vi "InitiateEventDisplay.vi"(6 "error in":errorcluster, 7 "colors":T1={"Frame color"=0, "Connectors color"=0, "Supports color"=0, "Bolts color"=0, "Scintillators color"=0, "Scintillator alpha"=0.5}, 8 "Scale":sgl, 9 "Path to detector WRL file":path) -> (0 "error out":errorcluster, 3 "Event Display Scene":refnum<vi>)   [LabVIEW 2016]
uses:
  <vilib>/picture/3D Picture Control/Object/Create Object (name).vi
  <vilib>/picture/3D Picture Control/NI_3D Picture Control.lvlib
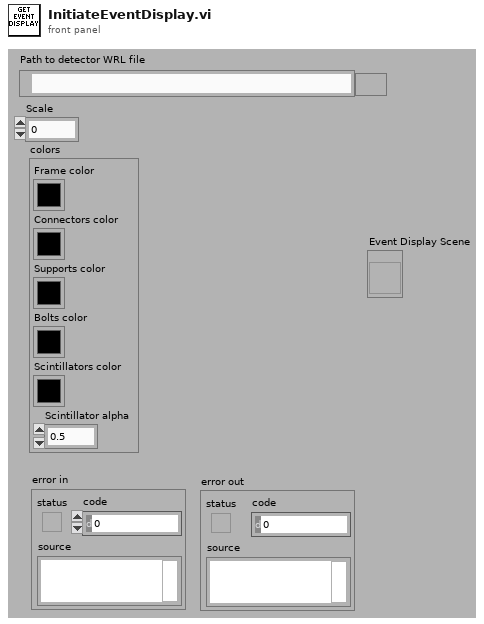
[diagram p1: front panel]
types:
  T1 = cluster{"Frame color":u32, "Connectors color":u32, "Supports color":u32, "Bolts color":u32, "Scintillators color":u32, "Scintillator alpha":sgl}
  T2 = enum16{"Normal Bin", "Opaque Bin", "Transparent Bin"}
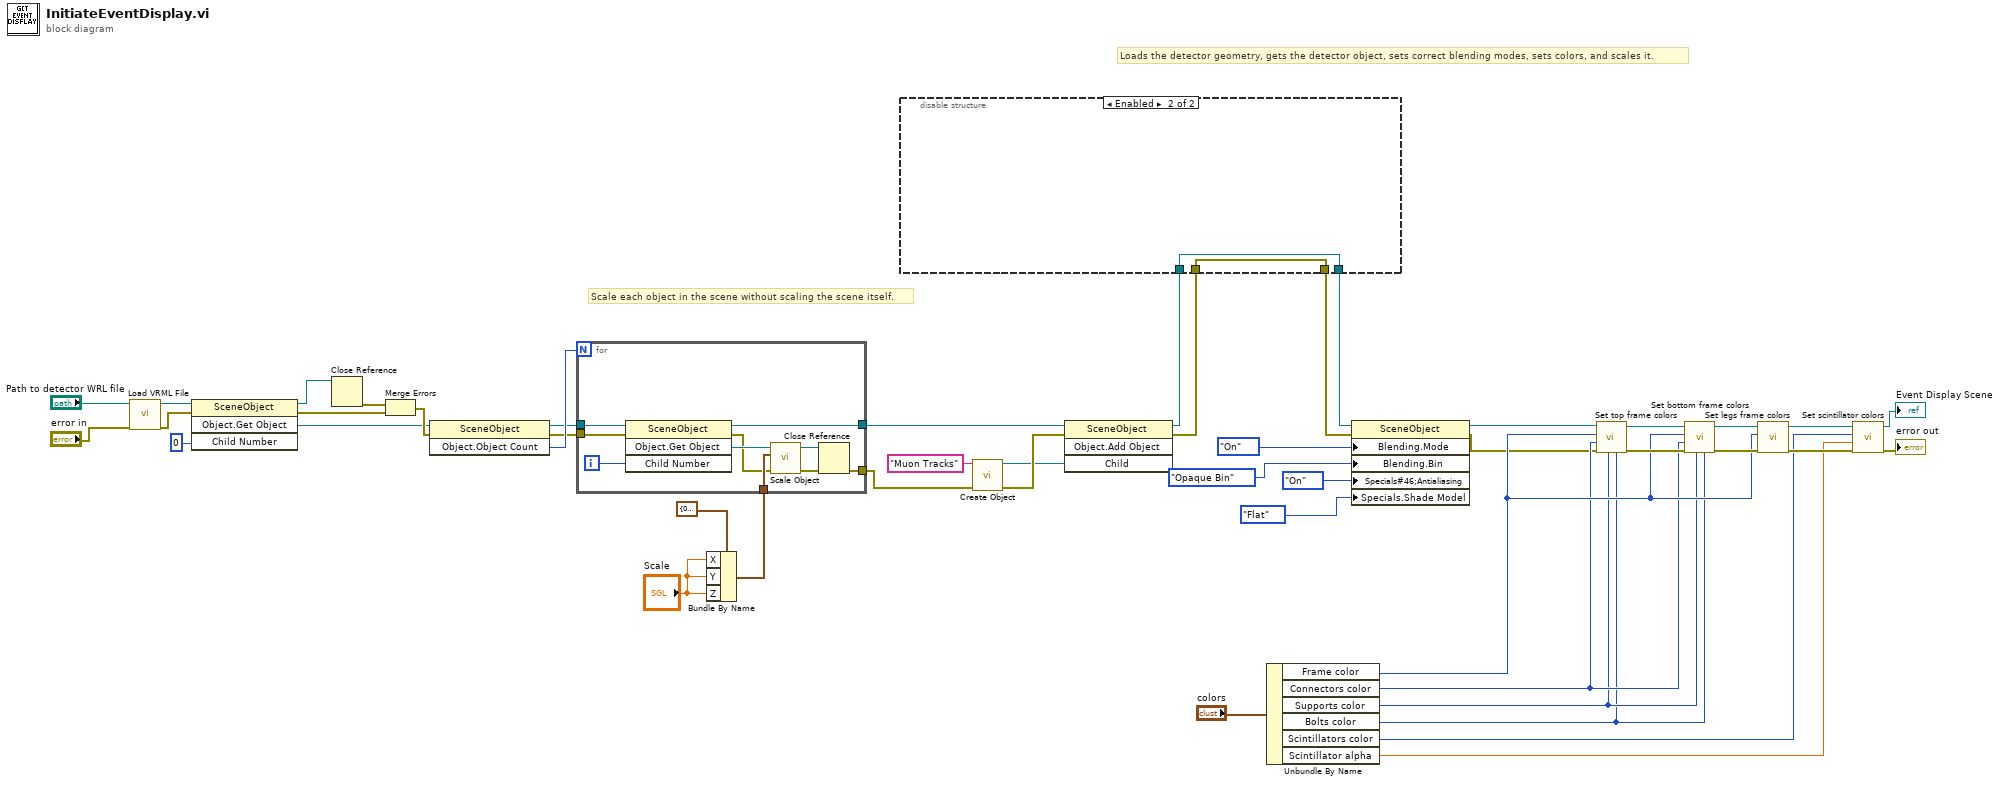
[diagram p0: block diagram]
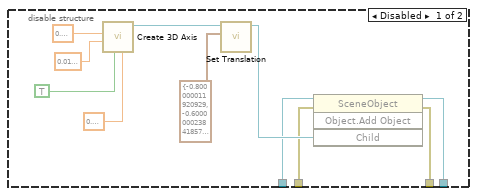
[diagram p2: hidden frame]
diagram:
  # "Scale each object in the scene without scaling the scene itself."
  # "Loads the detector geometry, gets the detector object, sets correct blending modes, sets colors, and scales it."
  n1 = call <vilib>:"Load VRML File.vi"("error in"="error in", "Path"="Path to detector WRL file") -> ("error out"=w26:errorcluster, "Scene:Read Scene File"=w45:refnum<vi>)  [unwired: 8 in]
  n2 = invoke class="SceneObject" method="Object.Get Object"(reference=w45, error in=w26, "Child Number"=0 ("index")) -> (reference out=w24:refnum<vi>, error out=w22:errorcluster, "Get Child"=w14:refnum<vi>)  [unwired: 1 in, 1 out]
  n3 = Close Reference(reference=w24) -> (error out=w23:errorcluster)  [unwired: 1 in]
  n4 = Merge Errors(w23, w22) -> (w15:errorcluster)
  n5 = invoke class="SceneObject" method="Object.Object Count"(reference=w14, error in=w15) -> (reference out=w12:refnum<vi>, error out=w11:errorcluster, "Child Count"=w13:i32)  [unwired: 1 in]
  n6 = Bundle By Name(cluster=cluster{"X":sgl, "Y":sgl, "Z":sgl} {"X"=0.0, "Y"=0.0, "Z"=0.0} ("Scale"), "X"="Scale", "Y"="Scale", "Z"="Scale") -> (w10:cluster{"X":sgl, "Y":sgl, "Z":sgl})
  n7 = for {
    N: w13 -> [_]
    tunnel: w12 -> [w56]
    tunnel: w11 -> [w55]
    tunnel: w10 -> [w52]
    tunnel: [w48] -> w9
    tunnel: [w47] -> w8
    i -> [w54]
    n8 = invoke class="SceneObject" method="Object.Get Object"(reference=w56, error in=w55, "Child Number"=w54) -> (reference out=w48:refnum<vi>, error out=w51:errorcluster, "Get Child"=w53:refnum<vi>)  [unwired: 1 in, 1 out]
    n9 = call <vilib>:"Scale Object.vi"("error in (no error)"=w51, "Scale"=w52, "Scene.Object In"=w53) -> ("error out"=w50:errorcluster, "Scene.Object Out"=w49:refnum<vi>)  [unwired: 7 in]
    n10 = Close Reference(reference=w49, error in (no error)=w50) -> (error out=w47:errorcluster)
  }
  n11 = call-poly <vilib>:"Create Object.vi"("error in (no error)"=w8, "Name"="Muon Tracks") -> ("error out"=w19:errorcluster, "Scene:New Object"=w5:refnum<vi>)  [unwired: 8 in]
  n12 = invoke class="SceneObject" method="Object.Add Object"(reference=w9, error in=w19, "Child"=w5) -> (reference out=w4:refnum<vi>, error out=w2:errorcluster)  [unwired: 1 in, 2 out]
  n13 = disable-structure shown="Enabled" {
    disable-tunnel: w4 -> [w60 w68]
    disable-tunnel: [w59 w68] -> w3
    disable-tunnel: w2 -> [w58 w69]
    disable-tunnel: [w57 w69] -> w1
    frame Disabled {
      n14 = call <vilib>:"Create 3D Axis.vi"("Character Size"=sgl 0.2, "Axis label?"=TRUE, "Radius"=sgl 0.02, "Length"=sgl 0.3) -> ("New Object Refnum"=w63:refnum<vi>)  [unwired: 6 in, 1 out]
      n15 = call <vilib>:"Set Translation.vi"("Translation"=cluster{"X":sgl, "Y":sgl, "Z":sgl} {"X"=-0.8, "Y"=-0.6, "Z"=0.8}, "Scene Object"=w63) -> ("Translated Object"=w61:refnum<vi>)  [unwired: 8 in, 1 out]
      n16 = invoke class="SceneObject" method="Object.Add Object"(reference=w60, error in=w58, "Child"=w61) -> (reference out=w59:refnum<vi>, error out=w57:errorcluster)  [unwired: 1 in, 2 out]
    }
    frame Enabled {
    }
  }
  n17 = Unbundle By Name("colors") -> ("Frame color"=w33:u32, "Connectors color"=w32:u32, "Supports color"=w31:u32, "Bolts color"=w30:u32, "Scintillators color"=w29:u32, "Scintillator alpha"=w28:sgl)
  n18 = property class="SceneObject"(reference=w3, error in=w1, "Blending.Mode"=enum16{"Inherit Value", "Off", "On"}."On" ("Blending:Mode"), "Blending.Bin"=T2."Opaque Bin" ("Blending:Bin"), "Specials#46;Antialiasing"=enum16{"Inherit Value", "Off", "On"}."On" ("Specials:Anti-aliasing"), "Specials.Shade Model"=enum16{"Inherit Value", "Flat", "Smooth"}."Flat" ("Specials:Shade Model")) -> (reference out=w37:refnum<vi>, error out=w27:errorcluster)
  n19 = call "Set top frame colors.vi"("Bolts"=w30, "Supports"=w31, "error in (no error)"=w27, "Frame connectors"=w32, "Metal frame"=w33, "Detector ref in"=w37) -> ("error out"=w42:errorcluster, "Detector ref out"=w43:refnum<vi>)  [unwired: 4 in]
  n20 = call "Set bottom frame colors.vi"("Bolts"=w30, "Supports"=w31, "error in (no error)"=w42, "Frame connectors"=w32, "Metal frame"=w33, "Detector ref in"=w43) -> ("error out"=w40:errorcluster, "Detector ref out"=w41:refnum<vi>)  [unwired: 4 in]
  n21 = call "Set legs frame colors.vi"("error in (no error)"=w40, "Legs frame"=w33, "Detector ref in"=w41) -> ("error out"=w39:errorcluster, "Detector ref out"=w38:refnum<vi>)  [unwired: 7 in]
  n22 = call "Set scintillator colors.vi"("error in (no error)"=w39, "Base alpha"=w28, "Scintillators base color"=w29, "Detector ref in"=w38) -> ("error out"=→"error out":errorcluster, "Detector ref out"=→"Event Display Scene":refnum<vi>)  [unwired: 6 in]
